vi "svx_Polar_Draw_Annotation.vi"(0 "Polar Plot ref in":refnum<vi>, 1 "State in":T1={"Property Name"=[], "Container bounds"={"Width"=550, "Height"=250}, "Scale range"={"Maximum"=1.0, "Increment"=1.0}, "PointIdx"=0, "Marker list"=[], "Color settings"={"Arrow color"=16860, "Magnitude major grid"=13816530, "Magnitude minor grid"=16777216, "Phase grid"=13816530, "Phase scale marker text"=0}, "Magnitude scale name"="Magnitude", "Magnitude scale format string"="%#.2e", "MagnitudeScale:Visible"=TRUE, "MagnitudeScaleLabel:Visible"=TRUE, "PhaseScale:Visible"=TRUE, "Marker:Visible"=TRUE, "Cursor:Visible"=FALSE, "CursorName:Visible"=TRUE, "Autoscale"=TRUE, "Marker color"=16860, "Line color"=16711680, "Cursor color"=16711680, "Magnitude scale marker color"=0, "Plot.Line Style"=0, "Plot.Line Width"=0, "Plot.Point Style"=0, "Cursor.Line Style"=0, "Cursor.Line Width"=0, "Cursor.Point Style"=0, "Cursor.Style"=4, "Marker.Point Style"=2, "Point/fill color"=16711680, "Background color"=16777225, "Cursor name"="", "Cursor Release"=refnum, "Scale Range Change"=refnum, "data size(s)"=[], "Selectors:Visible"=TRUE, "Selector:ring Strings"={"Selector:Custom Strings"=FALSE, "Selector:Row Strings []"=[], "Selector:Column Strings []"=[], "User:Row Strings []"=[], "User:Column Strings []"=[]}, "Lock Cursor Info Position"=FALSE, "CursLoc"={"magnitude"=0.0, "phase"=0.0, "time/rev/RPM"=0.0}, "Plot Area:Position"={"Left"=0, "Top"=0}, "Plot Area:Size"={"Width"=0, "Height"=0}, "Marker.Style"=0, "Indication Arcs"=[], "Arc.Selector"=0, "customized marker"=[], "tree Width"=0, " Parents Tags"=[], "Children Tags"=[], "open?"=[], "index"=[{"row index"=0, "column index"=0}], "Label"="", "custom strings changed"=FALSE, "Owning VI"=refnum, "Legend BG color"=16777225, "Legend font color"=0, "column Width"=203, "attribute"=variant} caption="State", 5 "position array":cluster{dbl, dbl}[](array[cluster]), 7 "Annotation Values":dbl[](array[numeric]), 9 "precision (6)":i16=3) -> (3 "State out":T1={"Property Name"=[], "Container bounds"={"Width"=550, "Height"=250}, "Scale range"={"Maximum"=1.0, "Increment"=1.0}, "PointIdx"=0, "Marker list"=[], "Color settings"={"Arrow color"=16860, "Magnitude major grid"=13816530, "Magnitude minor grid"=16777216, "Phase grid"=13816530, "Phase scale marker text"=0}, "Magnitude scale name"="Magnitude", "Magnitude scale format string"="%#.2e", "MagnitudeScale:Visible"=TRUE, "MagnitudeScaleLabel:Visible"=TRUE, "PhaseScale:Visible"=TRUE, "Marker:Visible"=TRUE, "Cursor:Visible"=FALSE, "CursorName:Visible"=TRUE, "Autoscale"=TRUE, "Marker color"=16860, "Line color"=16711680, "Cursor color"=16711680, "Magnitude scale marker color"=0, "Plot.Line Style"=0, "Plot.Line Width"=0, "Plot.Point Style"=0, "Cursor.Line Style"=0, "Cursor.Line Width"=0, "Cursor.Point Style"=0, "Cursor.Style"=4, "Marker.Point Style"=2, "Point/fill color"=16711680, "Background color"=16777225, "Cursor name"="", "Cursor Release"=refnum, "Scale Range Change"=refnum, "data size(s)"=[], "Selectors:Visible"=TRUE, "Selector:ring Strings"={"Selector:Custom Strings"=FALSE, "Selector:Row Strings []"=[], "Selector:Column Strings []"=[], "User:Row Strings []"=[], "User:Column Strings []"=[]}, "Lock Cursor Info Position"=FALSE, "CursLoc"={"magnitude"=0.0, "phase"=0.0, "time/rev/RPM"=0.0}, "Plot Area:Position"={"Left"=0, "Top"=0}, "Plot Area:Size"={"Width"=0, "Height"=0}, "Marker.Style"=0, "Indication Arcs"=[], "Arc.Selector"=0, "customized marker"=[], "tree Width"=0, " Parents Tags"=[], "Children Tags"=[], "open?"=[], "index"=[{"row index"=0, "column index"=0}], "Label"="", "custom strings changed"=FALSE, "Owning VI"=refnum, "Legend BG color"=16777225, "Legend font color"=0, "column Width"=203, "attribute"=variant} caption="State", 4 "Polar Plot ref out":refnum<vi>, 6 "AnntList":T4)   [LabVIEW 2017, in "SVX Polar Plot.xctl"]
uses:
  <vilib>/addons/_XControls/Polar Plot/SVX Polar Plot.xctl
  <vilib>/addons/_XControls/Polar Plot/subVIs/svx_Polar_Plot_Internal_State.ctl
  <vilib>/addons/_XControls/Polar Plot/subVIs/svx_Polar_Indication_Arcs.ctl
  <vilib>/addons/_XControls/Polar Plot/subVIs/svx_Polar_Customized_Markers.ctl
  <vilib>/Utility/miscctls.llb/LVAnnotationListTypeDef.ctl
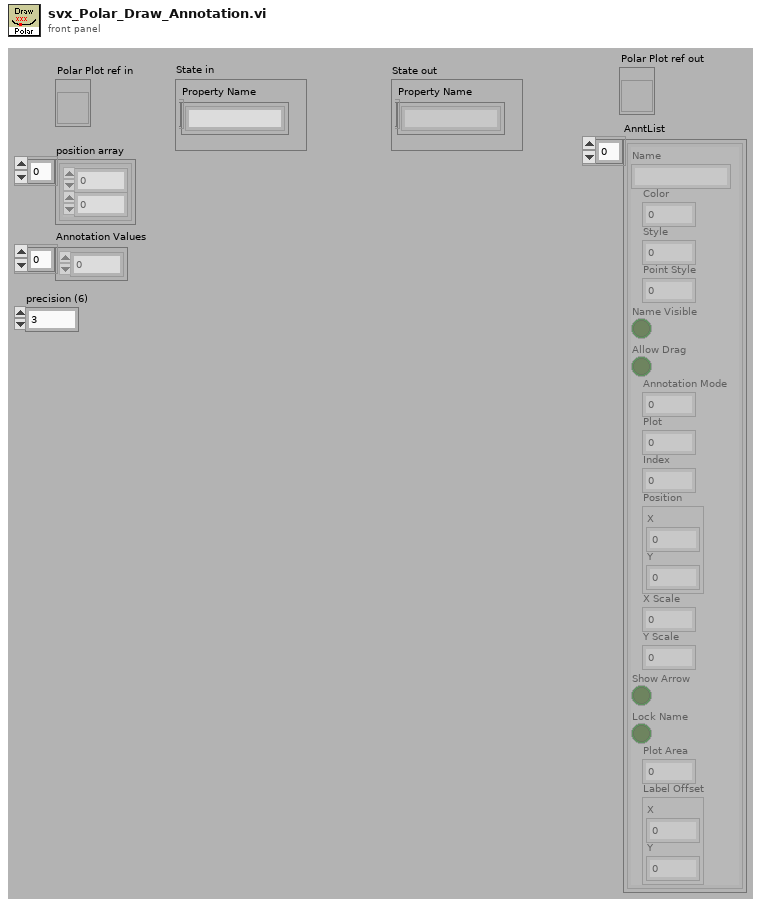
[diagram p1: front panel]
types:
  T1 = typedef "SVX Polar Plot.xctl/svx_Polar_Plot_Internal_State.ctl" = cluster{"Property Name":string[], "Container bounds":cluster{"Width":u32, "Height":u32}, "Scale range":cluster{"Maximum":dbl, "Increment":dbl}, "PointIdx":i32, "Marker list":cluster{"Name":string, "Color":u32, "Style":u8, "Point Style":u8, "Name Visible":bool, "Allow Drag":bool, "Annotation Mode":u32, "Plot":i32, "Index":i32, "Position":cluster{"X":dbl, "Y":dbl}, "X Scale":u32, "Y Scale":u32, "Show Arrow":bool, "Lock Name":bool, "Plot Area":i32, "Label Offset":cluster{"X":dbl, "Y":dbl}}[], "Color settings":cluster{"Arrow color":u32, "Magnitude major grid":u32, "Magnitude minor grid":u32, "Phase grid":u32, "Phase scale marker text":u32}, "Magnitude scale name":string, "Magnitude scale format string":string, "MagnitudeScale:Visible":bool, "MagnitudeScaleLabel:Visible":bool, "PhaseScale:Visible":bool, "Marker:Visible":bool, "Cursor:Visible":bool, "CursorName:Visible":bool, "Autoscale":bool, "Marker color":u32, "Line color":u32, "Cursor color":u32, "Magnitude scale marker color":u32, "Plot.Line Style":i32, "Plot.Line Width":i32, "Plot.Point Style":i32, "Cursor.Line Style":i32, "Cursor.Line Width":i32, "Cursor.Point Style":i32, "Cursor.Style":i32, "Marker.Point Style":i32, "Point/fill color":u32, "Background color":u32, "Cursor name":string, "Cursor Release":refnum<user-event>, "Scale Range Change":refnum<user-event>, "data size(s)":i32[], "Selectors:Visible":bool, "Selector:ring Strings":cluster{"Selector:Custom Strings":bool, "Selector:Row Strings []":string[], "Selector:Column Strings []":string[], "User:Row Strings []":string[], "User:Column Strings []":string[]}, "Lock Cursor Info Position":bool, "CursLoc":cluster{"magnitude":dbl, "phase":dbl, "time/rev/RPM":dbl}, "Plot Area:Position":cluster{"Left":i32, "Top":i32}, "Plot Area:Size":cluster{"Width":u32, "Height":u32}, "Marker.Style":i32, "Indication Arcs":T2, "Arc.Selector":u16, "customized marker":T3, "tree Width":u32, " Parents Tags":string[], "Children Tags":string[], "open?":bool[], "index":cluster{"row index":i32, "column index":i32}[], "Label":string, "custom strings changed":bool, "Owning VI":refnum<vi>, "Legend BG color":u32, "Legend font color":u32, "column Width":u32, "attribute":variant}
  T2 = typedef "SVX Polar Plot.xctl/svx_Polar_Indication_Arcs.ctl" = cluster{"Name":string, "Start radius":dbl, "End radius":dbl, "Line Style":i32, "Line Width":i32, "Border color":u32, "Fill color":u32, "Start angle":i16, "End angle":i16, "Visible":bool}[]
  T3 = typedef "SVX Polar Plot.xctl/svx_Polar_Customized_Markers.ctl" = cluster{"Name":string, "Color":u32, "Style":u8, "Point Style":u8, "Name Visible":bool, "Allow Drag":bool, "Annotation Mode":u32, "Plot":i32, "Index":i32, "Position":cluster{"Magnitude":dbl, "Phase":dbl}, "X Scale":u32, "Y Scale":u32, "Show Arrow":bool, "Lock Name":bool, "Plot Area":i32, "Label Offset":cluster{"Magnitude":dbl, "Phase":dbl}}[]
  T4 = typedef "LVAnnotationListTypeDef.ctl" = cluster{"Name":string, "Color":u32, "Style":u8, "Point Style":u8, "Name Visible":bool, "Allow Drag":bool, "Annotation Mode":u32, "Plot":i32, "Index":i32, "Position":cluster{"X":dbl, "Y":dbl}, "X Scale":u32, "Y Scale":u32, "Show Arrow":bool, "Lock Name":bool, "Plot Area":i32, "Label Offset":cluster{"X":dbl, "Y":dbl}}[]
  T5 = cluster{"Name":string, "Color":u32, "Style":u8, "Point Style":u8, "Name Visible":bool, "Allow Drag":bool, "Annotation Mode":u32, "Plot":i32, "Index":i32, "Position":cluster{"X":dbl, "Y":dbl}, "X Scale":u32, "Y Scale":u32, "Show Arrow":bool, "Lock Name":bool, "Plot Area":i32, "Label Offset":cluster{"X":dbl, "Y":dbl}}
  T6 = cluster{"Name":string, "Color":u32, "Style":u8, "Point Style":u8, "Name Visible":bool, "Allow Drag":bool, "Annotation Mode":u32, "Plot":i32, "Index":i32, "Position":cluster{"X":dbl, "Y":dbl}, "X Scale":u32, "Y Scale":u32, "Show Arrow":bool, "Lock Name":bool, "Plot Area":i32, "Label Offset":cluster{"X":dbl, "Y":dbl}}[]
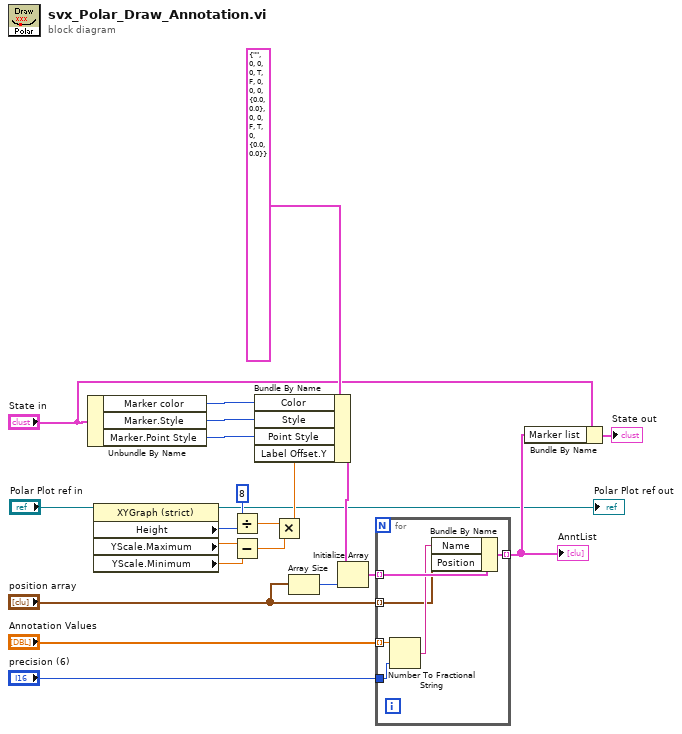
[diagram p0: block diagram]
diagram:
  n1 = Unbundle By Name("State in") -> ("Marker color"=w8:u32, "Marker.Style"=w7:i32, "Marker.Point Style"=w6:i32)
  n2 = property class="XYGraph (strict)"(reference="Polar Plot ref in") -> (reference out=→"Polar Plot ref out":refnum<vi>, "Height"=w16:u32, "YScale.Maximum"=w14:dbl, "YScale.Minimum"=w13:dbl)  [unwired: 1 in, 1 out]
  n3 = Divide(x=u32 8, y=w16) -> (x/y=w12:dbl)
  n4 = Subtract(x=w14, y=w13) -> (x-y=w11:dbl)
  n5 = Multiply(x=w12, y=w11) -> (x*y=w9:dbl)
  n6 = Bundle By Name(cluster=T5 {"Name"="", "Color"=0, "Style"=0, "Point Style"=0, "Name Visible"=TRUE, "Allow Drag"=FALSE, "Annotation Mode"=0, "Plot"=0, "Index"=0, "Position"={"X"=0.0, "Y"=0.0}, "X Scale"=0, "Y Scale"=0, "Show Arrow"=FALSE, "Lock Name"=TRUE, "Plot Area"=0, "Label Offset"={"X"=0.0, "Y"=0.0}}, "Color"=w8, "Style"=w7, "Point Style"=w6, "Label Offset.Y"=w9) -> (w17:T5)
  n7 = Array Size(array="position array") -> (size(s)=w18:i32)
  n8 = Initialize Array(w17, w18) -> (w10:T6)
  n9 = for {
    tunnel: "Annotation Values" -> [w28] mode=indexing
    tunnel: "precision (6)" -> [w27]
    tunnel: "position array" -> [w24] mode=indexing
    tunnel: w10 -> [w26] mode=indexing
    tunnel: [w23] -> w4 mode=indexing
    n10 = Number To Fractional String(number=w28, precision (6)=w27) -> (F-format string=w25:string)  [unwired: 2 in]
    n11 = Bundle By Name(cluster=w26, "Name"=w25, "Position"=w24) -> (w23:T5)
  }
  "AnntList" <- w4
  n12 = Bundle By Name(cluster="State in", "Marker list"=w4) -> (→"State out":T1)
